vi "TimerTest.vi"() -> ()   [LabVIEW 2015]
panel:
  in  "stop":bool
  out "E":bool
  in  "OK Button":bool
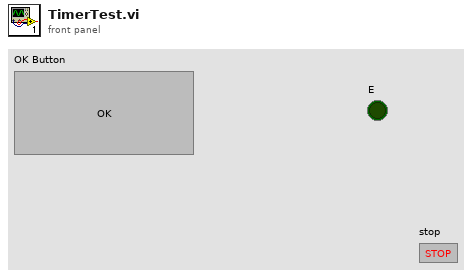
[diagram p1: front panel]
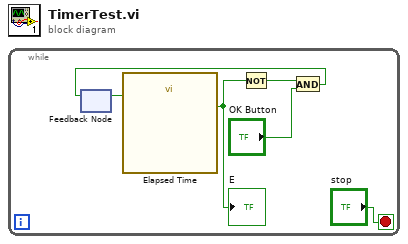
[diagram p0: block diagram]
diagram:
  n1 = while {
    stop <- "stop" stop-if-true
    n2 = feedback #1() -> (w2:bool)  [unwired: 1 in]
    n3 = call "Elapsed Time"("Reset"=w2) -> ("Time has Elapsed"=w5:bool)  [unwired: 11 in, 7 out]
    "E" <- w5
    n4 = Not(x=w5) -> (.not. x?=w4:bool)
    n5 = And(x=w4, y="OK Button") -> (x .and. y?=w3:bool)
    n6 = feedback-in #1(w3) -> ()
  }
